vi "N_Rayleigh_Flow Model (SubVI).vi"(4 "EDQ (ml/s)":dbl, 5 "PSQ (ml/s)":dbl, 7 "T_Flow Start":dbl, 8 "Parameters (1XN)":dbl[](array[numeric])=[0.01, 0.02], 9 "Pressure (mmHg)":waveform(dbl)) -> (0 "Waveform Graph":dbl[][](graph), 3 "n-Rayleigh Model Flow":waveform(dbl))   [LabVIEW 2017]
doc: "This template is the starting point for creating a model function to be passed to the Nonlinear Curve Fit.vi."
uses:
  <vilib>/Analysis/NI_AALBase.lvlib
  <vilib>/Analysis/1siggen.llb/Ramp Pattern by Delta.vi
panel:
  out "Waveform Graph 2":dbl[](graph)
  out "size(s)":i32
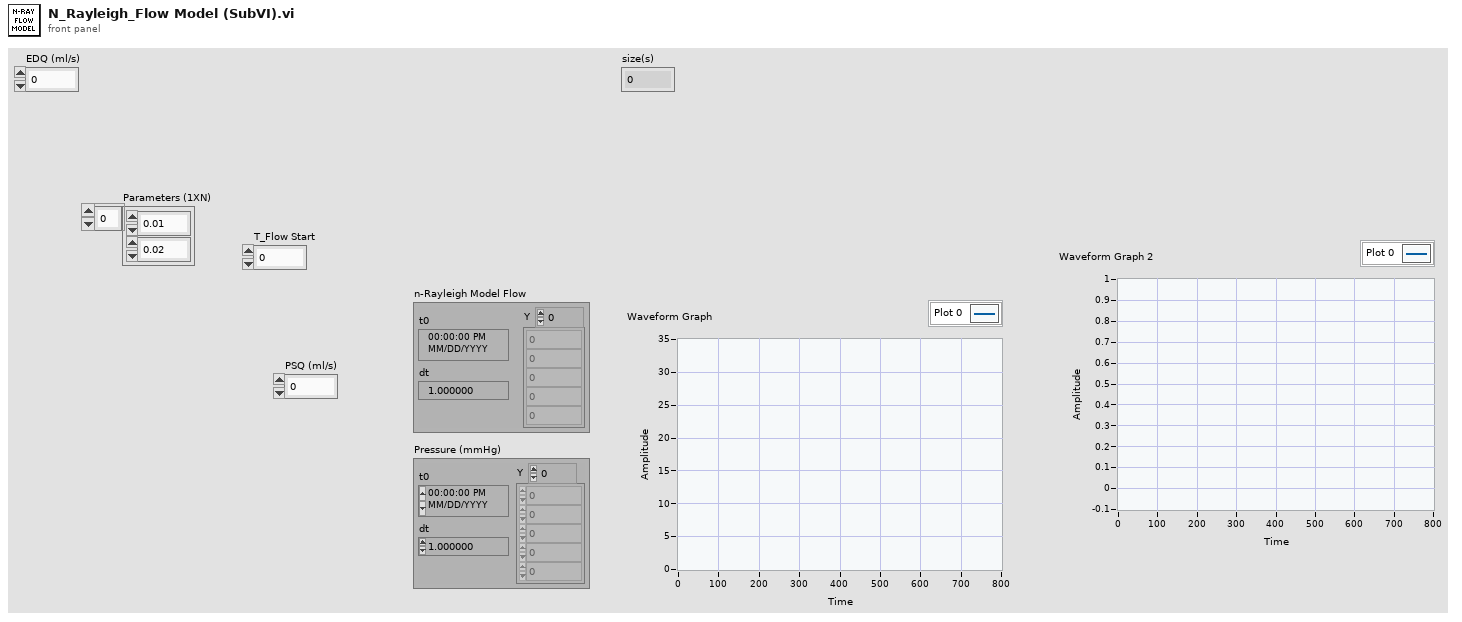
[diagram p1: front panel]
types:
  T1 = enum32{"Lowpass", "Highpass", "Bandpass", "Bandstop"}
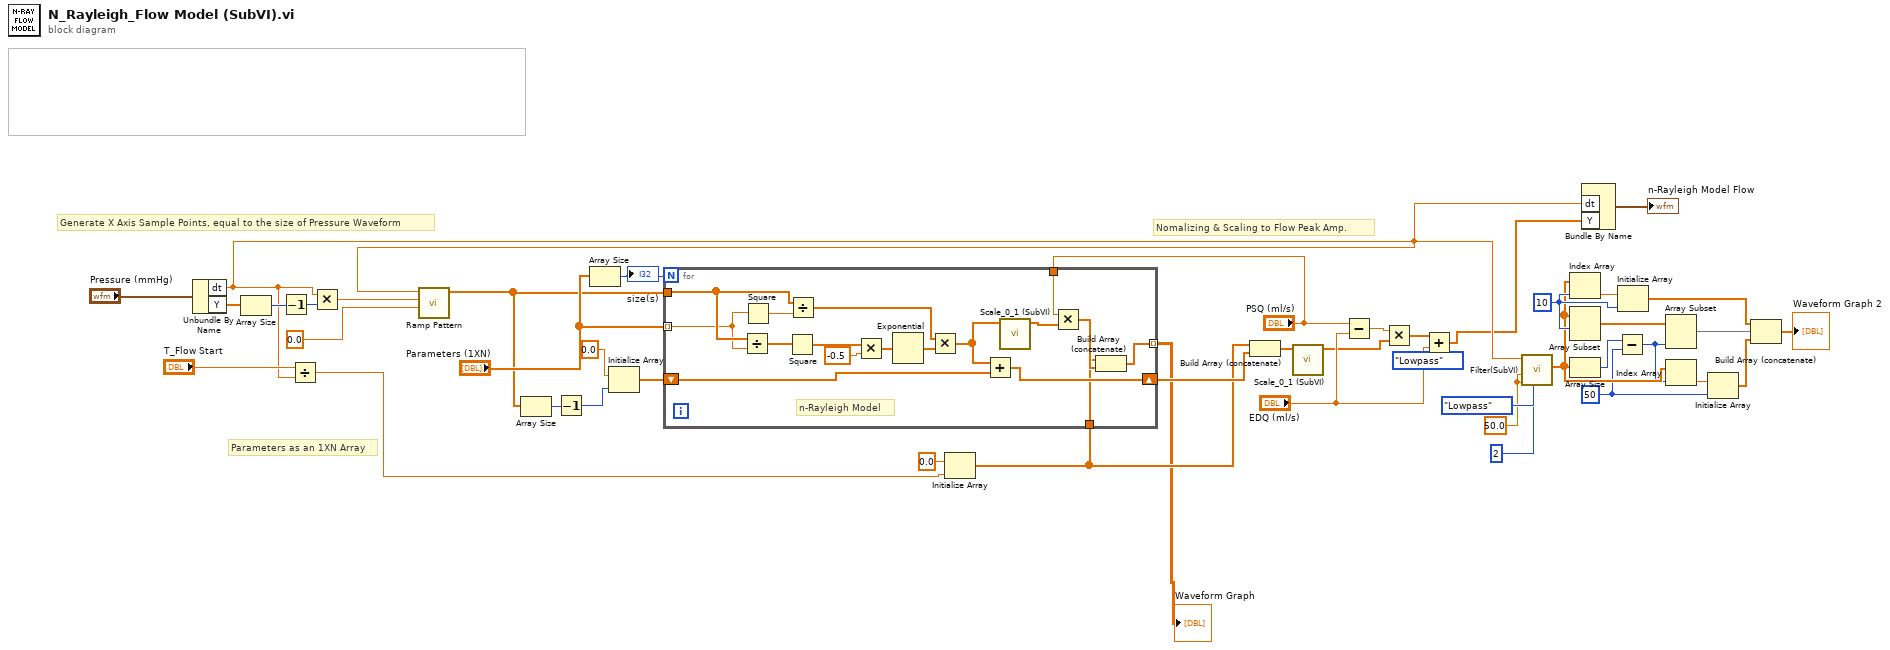
[diagram p0: block diagram]
diagram:
  w9 = 50 ("y")
  w14 = 10 ("index")
  w17 = 50.0 ("high cutoff freq: fh")
  (unwired) T1."Lowpass" ("filter type")
  # "Nomalizing & Scaling to Flow Peak Amp."
  # "Parameters as an 1XN Array"
  # "Generate X Axis Sample Points, equal to the size of Pressure Waveform"
  n1 = Unbundle By Name("Pressure (mmHg)") -> ("dt"=w16:dbl, "Y"=w43:dbl[])
  n2 = Array Size(array=w43) -> (size(s)=w39:i32)
  n3 = Decrement(x=w39) -> (x-1=w40:i32)
  n4 = Divide ("(x-b1)/c")(x="T_Flow Start", y=w16) -> (x/y=w30:dbl)
  n5 = Multiply(x=w16, y=w40) -> (x*y=w41:dbl)
  n6 = call-poly <vilib>:"Ramp Pattern.vi"("start"=0.0 ("element"), "end"=w41, "delta"=w16) -> ("Ramp Pattern"=w34:dbl[])  [unwired: 6 in, 2 out]
  n7 = Array Size(array=w34) -> (size(s)=w33:i32)
  n8 = Decrement(x=w33) -> (x-1=w32:i32)
  n9 = Array Size(array="Parameters (1XN)") -> (size(s)=w36:i32)
  "size(s)" <- w36
  n10 = Initialize Array(0.0 ("element"), w32) -> (w37:dbl[])
  n11 = Initialize Array(0.0 ("element"), w30) -> (w24:dbl[])
  n12 = for {
    N: w36 -> [_]
    tunnel: w34 -> [w59]
    shift-right: [w50] -> w29
    shift-left: w37 -> [w52]
    tunnel: "Parameters (1XN)" -> [w51] mode=indexing
    tunnel: [w44] -> w2 mode=indexing
    tunnel: "PSQ (ml/s)" -> [w47]
    tunnel: w24 -> [w45]
    # "n-Rayleigh Model"
    n13 = Divide ("(x-b1)/c")(x=w59, y=w51) -> (x/y=w53:dbl[])
    n14 = Square(x=w51) -> (x^2=w57:dbl)
    n15 = Square(x=w53) -> (x^2=w55:dbl[])
    n16 = Divide ("(x-b1)/c")(x=w59, y=w57) -> (x/y=w60:dbl[])
    n17 = Multiply(x=w55, y=-0.5) -> (x*y=w54:dbl[])
    n18 = Exponential(1:w54) -> (0:w56:dbl[])
    n19 = Multiply(x=w60, y=w56) -> (x*y=w49:dbl[])
    n20 = Add(x=w49, y=w52) -> (x+y=w50:dbl[])
    n21 = call "Scale_0_1 (SubVI).vi"("BLine D"=w49) -> ("Array"=w48:dbl[])  [unwired: 10 in]
    n22 = Multiply(x=w47, y=w48) -> (x*y=w46:dbl[])
    n23 = Build Array (concatenate)(w45, w46) -> (w44:dbl[])
  }
  "Waveform Graph" <- w2
  n24 = Build Array (concatenate)(w24, w29) -> (w28:dbl[])
  n25 = call "Scale_0_1 (SubVI).vi"("BLine D"=w28) -> ("Array"=w1:dbl[])  [unwired: 10 in]
  n26 = Subtract(x="PSQ (ml/s)", y="EDQ (ml/s)") -> (x-y=w22:dbl)
  n27 = Multiply(x=w22, y=w1) -> (x*y=w21:dbl[])
  n28 = Add(x=w21, y="EDQ (ml/s)") -> (x+y=w13:dbl[])
  n29 = call "Filter(SubVI).vi"("order"=2, "filter type"=T1."Lowpass", "low cutoff freq: fl"=w17, "high cutoff freq: fh"=w17, "dt"=w16) -> ("Filtered Data"=w11:dbl[])  [unwired: 6 in]
  n30 = Index Array(array=w11, index=w14) -> (element=w12:dbl)
  n31 = Array Subset(array=w11, index=w14) -> (w5:dbl[])  [unwired: 1 in]
  n32 = Array Size(array=w11) -> (size(s)=w15:i32)
  n33 = Bundle By Name("dt"=w16, "Y"=w13) -> (→"n-Rayleigh Model Flow":waveform(dbl))  [unwired: 1 in]
  n34 = Subtract(x=w15, y=w9) -> (x-y=w8:i32)
  n35 = Initialize Array(w12, w14) -> (w4:dbl[])
  n36 = Array Subset(array=w5, length=w8) -> (w7:dbl[])  [unwired: 1 in]
  n37 = Index Array(array=w11, index=w8) -> (element=w10:dbl)
  n38 = Initialize Array(w10, w9) -> (w6:dbl[])
  n39 = Build Array (concatenate)(w4, w7, w6) -> (→"Waveform Graph 2":dbl[])
